vi "Splite string AC_PC_SC.vi"() -> ()   [LabVIEW 2017]
panel:
  out "spreadsheet string":string
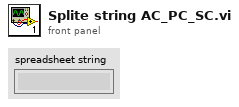
[diagram p1: front panel]
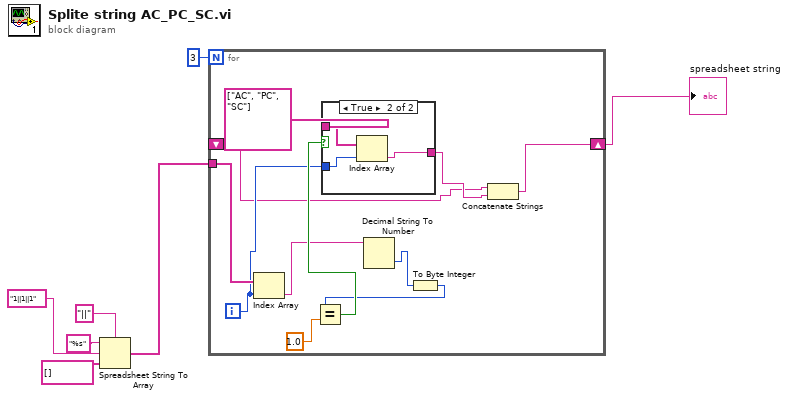
[diagram p0: block diagram]
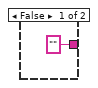
[diagram p2: hidden frame]
diagram:
  n1 = Spreadsheet String To Array(delimiter (Tab)="||", format string="%s", spreadsheet string="1||1||1", array type (2D Dbl)=string[] []) -> (array=w2:string[])
  n2 = for {
    N: 3 -> [_]
    tunnel: w2 -> [w18]
    shift-right: [w10] -> w1
    shift-left: _ -> [w8]
    i -> [w14]
    n3 = Index Array(array=w18, index=w14) -> (element=w13:string)
    n4 = Decimal String To Number(string=w13) -> (number=w12:i32)  [unwired: 2 in, 1 out]
    n5 = To Byte Integer(number=w12) -> (8bit integer=w11:i8)
    n6 = Equal?(x=w11, y=1.0) -> (x = y?=w16:bool)
    n7 = case shown="True" w16 {
      tunnel: string[] ["AC", "PC", "SC"] -> [_ w22]
      tunnel: w14 -> [_ w21]
      tunnel: ["" ("String") w20] -> w9
      frame False {
      }
      frame True {
        n8 = Index Array(array=w22, index=w21) -> (element=w20:string)
      }
    }
    n9 = Concatenate Strings(w8, w9) -> (w10:string)
  }
  "spreadsheet string" <- w1
